vi "preform rotate op -numeric.vi"(8 "error in (no error)":errorcluster, 10 "Face to act on":u8, 11 "Rotate command":T2=enum."Middle row left") -> (0 "error out(no error)":errorcluster, 2 "Facets To move":T1[](array[typedef]), 3 "Axis":cluster{"X":sgl, "Y":sgl, "Z":sgl})   [LabVIEW 2019]
uses:
  Cube Data Ops.ctl
  Rubix Array data type.ctl
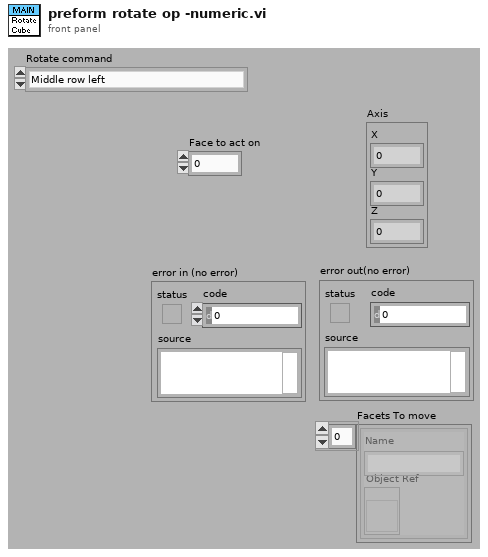
[diagram p1: front panel]
types:
  T1 = typedef "Rubix Array data type.ctl" = cluster{"Object Ref":refnum<vi>, "Name":string}
  T2 = typedef "Cube Data Ops.ctl" = enum16{"Initialize", "Set Rubix Ref Array", "Set Rubix Text Array", "Set Current Face", "Get Rubix Text Array", "Generate Rubix Array", "Get Rubix array", "Get Facets to move", "Randomize", "Top row left", "Top row right", "Middle row left", "Middle row right", "Bottom row left", "Bottom row right", "Left column up", "Left column down", "Middle column up", "Middle column down", "Right column up", "Right column down", "Face ccw", "Face cw"}
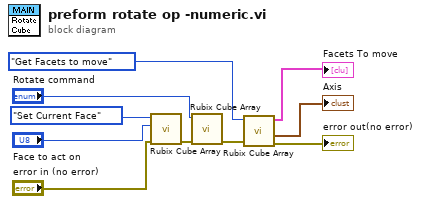
[diagram p0: block diagram]
diagram:
  n1 = call "Rubix Cube Array.vi"("error in (no error)"="error in (no error)", "Face to act on"="Face to act on", "Command"=Cube_Data_Ops."Set Current Face" ("Enum")) -> ("error out(no error)"=w9:errorcluster)  [unwired: 4 in, 4 out]
  n2 = call "Rubix Cube Array.vi"("error in (no error)"=w9, "Command"="Rotate command") -> ("error out(no error)"=w6:errorcluster)  [unwired: 5 in, 4 out]
  n3 = call "Rubix Cube Array.vi"("error in (no error)"=w6, "Command"=Cube_Data_Ops."Get Facets to move") -> ("error out(no error)"=→"error out(no error)":errorcluster, "Axis"=→"Axis":cluster{"X":sgl, "Y":sgl, "Z":sgl}, "Facets To move"=→"Facets To move":T1[])  [unwired: 5 in, 2 out]
